vi "full uart with motor control demo.vi"() -> ()   [LabVIEW 2018]
uses:
  <vilib>/Instr/_visa.llb/VISA Configure Serial Port (Instr).vi
panel:
  in  "speed 4":string
  in  "speed 3":string
  in  "speed 2":string
  in  "speed 1":string
  in  "Length of individual speed command (including sign)":i32=6
  in  "Number of Motors to control":i32=4
  out "All sppeds array (double)":dbl[](array[numeric])
  in  "timeout (10sec)":u32=10000
  in  "stop":bool
  # "Write the indivual speeds here, noting that you must include the\n+ sign for positive values, and - for negative values:\n\ne.g.\n+0.232\n-0.234\n+0.254\n-0.233"
  # "output"
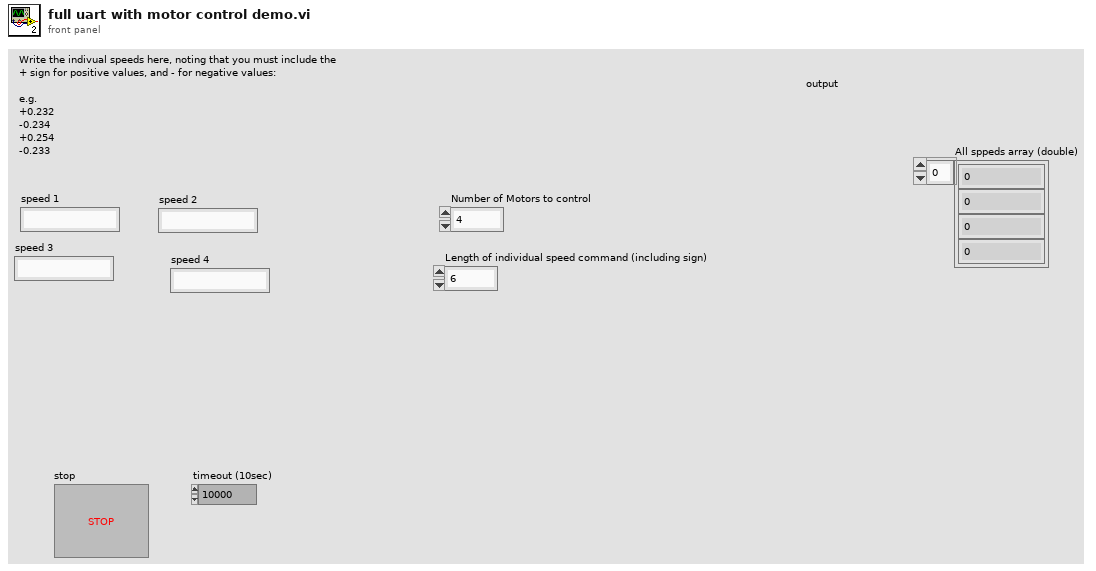
[diagram p1: front panel]
types:
  T1 = typedef "All Addresses.ctl" = u8[]
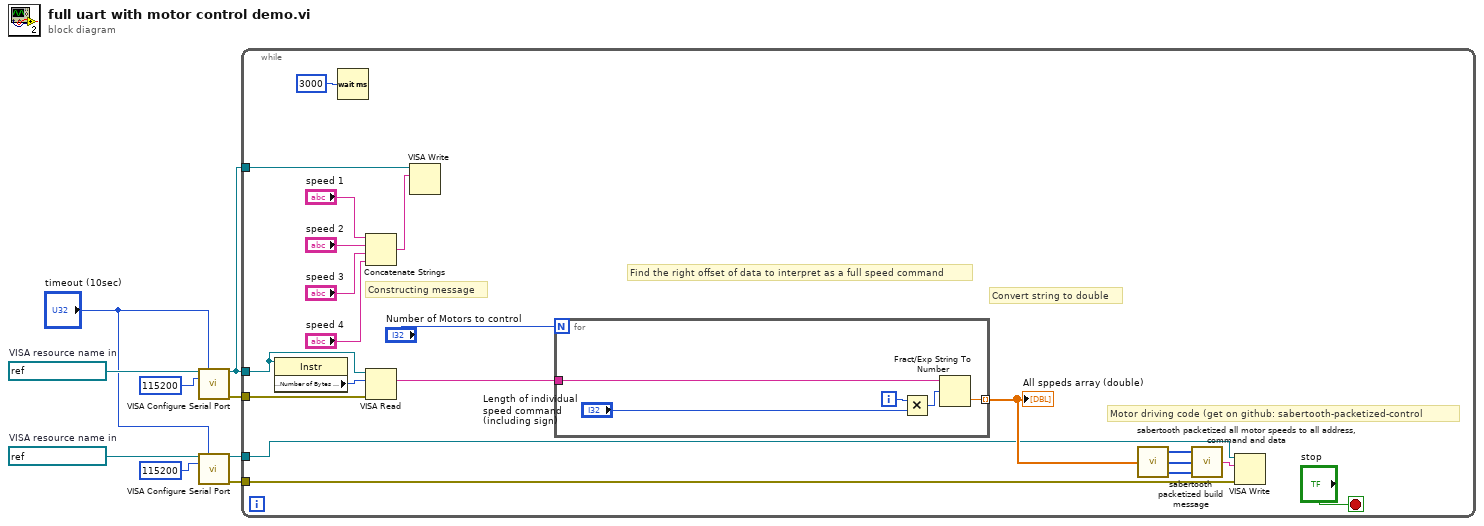
[diagram p0: block diagram]
diagram:
  w4 = refnum<visa-resource-name> "ASRL1::INSTR"  # VISA resource name in
  w9 = refnum<visa-resource-name> "ASRL2::INSTR"  # VISA resource name in
  n1 = call-poly "VISA Configure Serial Port"("VISA resource name"=w9, "timeout (10sec)"="timeout (10sec)", "baud rate (9600)"=u32 115200) -> ("VISA resource name out"=w7:refnum<visa-resource-name>, "error out"=w6:errorcluster)  [unwired: 11 in]
  n2 = call-poly "VISA Configure Serial Port"("VISA resource name"=w4, "timeout (10sec)"="timeout (10sec)", "baud rate (9600)"=u32 115200) -> ("VISA resource name out"=w2:refnum<visa-resource-name>, "error out"=w1:errorcluster)  [unwired: 11 in]
  n3 = while {
    tunnel: w7 -> [w28]
    tunnel: w7 -> [w26]
    tunnel: w6 -> [w25]
    tunnel: w2 -> [w12]
    tunnel: w1 -> [w10]
    stop <- "stop" stop-if-true
    # "Motor driving code (get on github: sabertooth-packetized-control"
    # "Convert string to double"
    # "Find the right offset of data to interpret as a full speed command"
    # "Constructing message"
    n4 = property class="Instr"(reference=w28) -> ("Serial Settings:Number of Bytes at Serial Port"=w27:u32)  [unwired: 1 in, 2 out]
    n5 = Wait (ms)(milliseconds to wait=u32 3000) -> ()  [unwired: 1 out]
    n6 = Concatenate Strings("speed 1", "speed 2", "speed 3", "speed 4") -> (w23:string)
    n7 = VISA Read(VISA resource name=w28, byte count=w27, error in (no error)=w25) -> (read buffer=w22:string)  [unwired: 3 out]
    n8 = VISA Write(VISA resource name=w26, write buffer=w23) -> ()  [unwired: 1 in, 3 out]
    n9 = for {
      N: "Number of Motors to control" -> [_]
      tunnel: [w34] -> w13 mode=indexing
      tunnel: w22 -> [w31]
      i -> [w30]
      n10 = Multiply(x=w30, y="Length of individual speed command (including sign)") -> (x*y=w33:i32)
      n11 = Fract/Exp String To Number(string=w31, offset=w33) -> (number=w34:dbl)  [unwired: 2 in, 1 out]
    }
    "All sppeds array (double)" <- w13
    n12 = call "sabertooth packetized all motor speeds to all address, command and data.vi"("All Motor Speeds"=w13) -> ("All Addresses"=w16:T1, "All Commands"=w15:u8[], "All Data"=w14:u8[])
    n13 = call "sabertooth packetized build message.vi"("All Data"=w14, "All Commands"=w15, "All Addresses"=w16) -> ("Uart Write Data"=w11:string)
    n14 = VISA Write(VISA resource name=w12, write buffer=w11, error in (no error)=w10) -> ()  [unwired: 3 out]
  }
